vi "Connect.vi"(5 "PQ Connection type":refnum<class "PQ Connection.lvclass">, 8 "error in (no error)":errorcluster, 10 "Connection Strings":string="host=localhost port=5432 dbname = mydb ") -> (0 "error out":errorcluster, 3 "PQ Connection out":refnum<class "PQ Connection.lvclass">)   [LabVIEW 2013, in "PQ Connection.lvclass"]
doc: "Opens a connection to the PostgreSQL database, as specified in the COnnection String.\n\nSee:\nhttps://www.postgresql.org/docs/9.6/static/libpq-connect.html#LIBPQ-CONNSTRING"
uses:
  PQ Connection.lvclass
  PQ Connection.lvclass/PQ Connection.ctl
  Error.vi
  libpq.dll
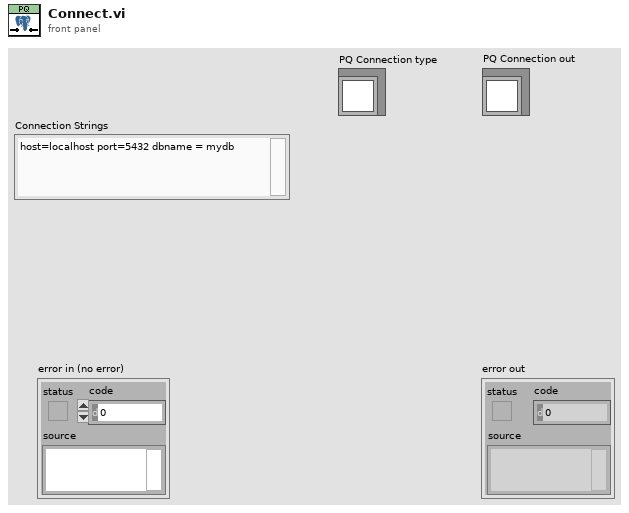
[diagram p1: front panel]
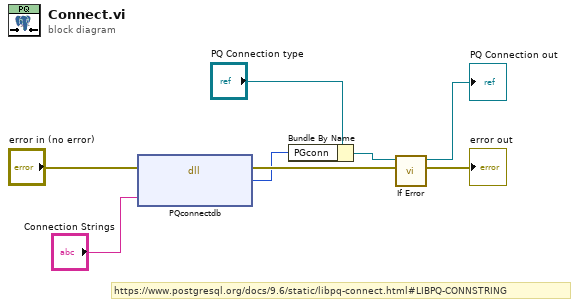
[diagram p0: block diagram]
diagram:
  # "https://www.postgresql.org/docs/9.6/static/libpq-connect.html#LIBPQ-CONNSTRING"
  n1 = dll-call lib="C:/Users/patrick/Documents/GitHub/Leiden-FP/src/Write to PGSQL/PostgreSQL Library/Connection/libpq.dll" fn="PQconnectdb"(error in="error in (no error)", "conninfo"="Connection Strings") -> (error out=w6:errorcluster, "PGconn"=w1:u32)  [unwired: 3 in, 1 out]
  n2 = Bundle By Name(cluster="PQ Connection type", "PGconn"=w1) -> (w2:refnum<class "PQ Connection.lvclass">)
  n3 = call "If Error.vi"("error in (no error)"=w6, "PQ Connection in"=w2) -> ("error out"=→"error out":errorcluster, "PQ Connection out"=→"PQ Connection out":refnum<class "PQ Connection.lvclass">)  [unwired: 8 in]
